vi "Untitled 1.vi"() -> ()   [LabVIEW 2019]
uses:
  Estados.ctl
panel:
  out "HANDLE":u32
  out "Error (\"1\" Error)":bool
  out "Todos":T1(array[cluster])=[{"Device Index"=0, "FT_FLAGS_OPENED"=TRUE, "FT_FLAGS_HISPEED"=TRUE, "Type"=6, "VID"=1027, "PID"=24592, "LocID"=1131585, "Serial Number"="CTAV2022A", "Description"="MI CTA TEST A", "FT_Handle"=433820616}, {"Device Index"=1, "FT_FLAGS_OPENED"=TRUE, "FT_FLAGS_HISPEED"=TRUE, "Type"=6, "VID"=1027, "PID"=24592, "LocID"=1131586, "Serial Number"="CTAV2022B", "Description"="MI CTA TEST B", "FT_Handle"=433822896}]
  out "Array CTA":T1(array[cluster])=[{"Device Index"=0, "FT_FLAGS_OPENED"=TRUE, "FT_FLAGS_HISPEED"=TRUE, "Type"=6, "VID"=1027, "PID"=24592, "LocID"=1131585, "Serial Number"="CTAV2022A", "Description"="MI CTA TEST A", "FT_Handle"=433820616}]
  out "Valor Asic":u16 format="%x"
  in  "error in (no error)":errorcluster
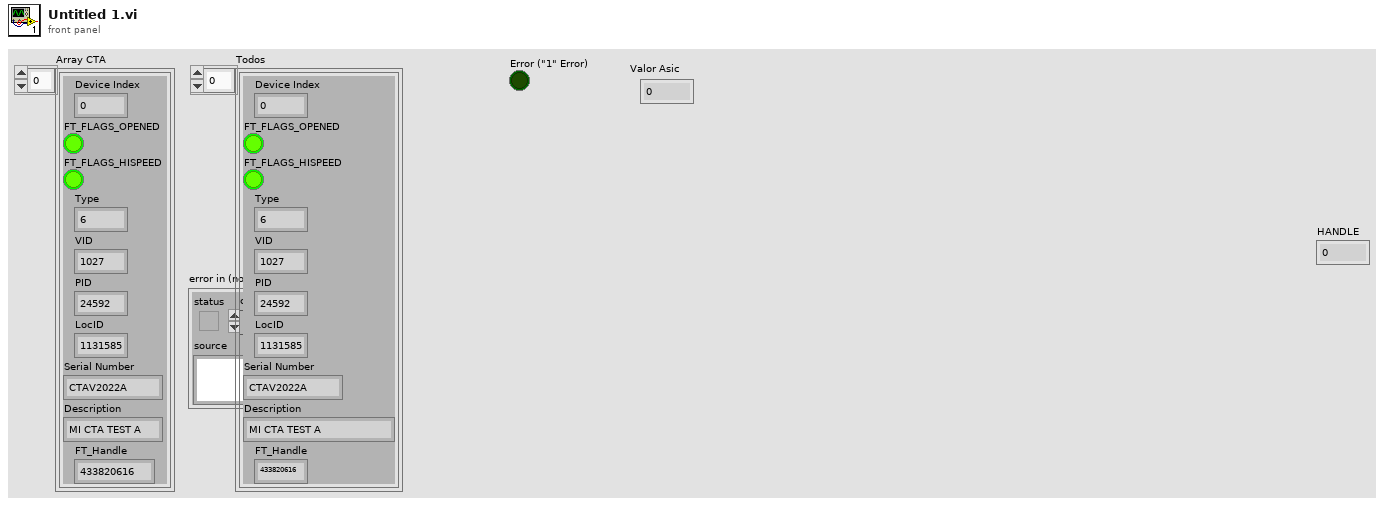
[diagram p1: front panel]
types:
  T1 = cluster{"Device Index":u32, "FT_FLAGS_OPENED":bool, "FT_FLAGS_HISPEED":bool, "Type":u32, "VID":u32, "PID":u32, "LocID":i32, "Serial Number":string, "Description":string, "FT_Handle":u32}[]
  T2 = typedef "Estados.ctl" = enum16{"Inicio", "FuenteON", "Espera", "FuenteOFF", "ObtenerHandle", "InitGen", "Fin", "RateScan", "CerrarVISA"}
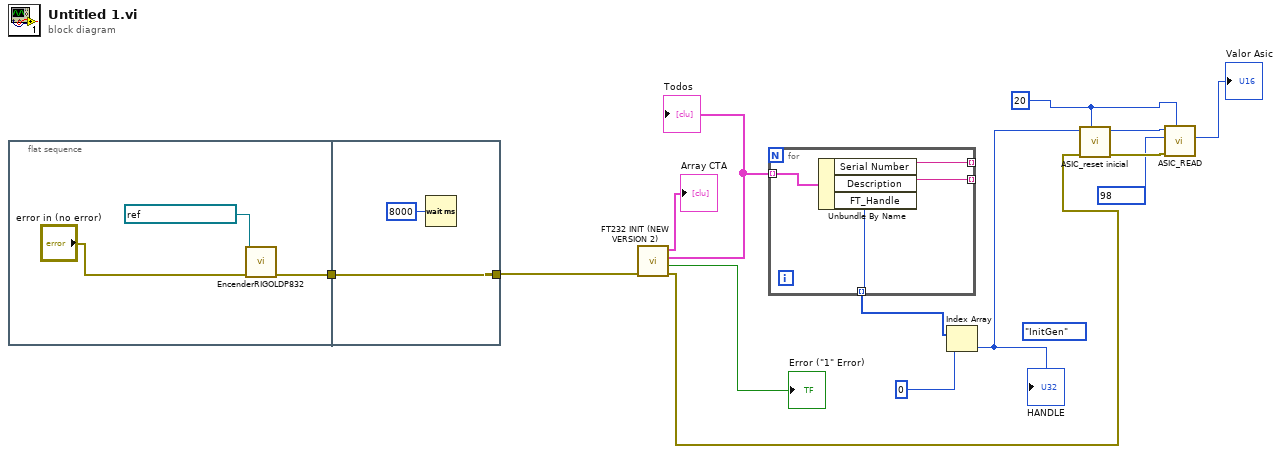
[diagram p0: block diagram]
diagram:
  (unwired) Estados."InitGen"
  w10 = u32 20 ("Espera acceso USB")
  n1 = flat-sequence {
    tunnel: [w15] -> w1
    tunnel: [w19] -> w2
    tunnel: w1 -> [w19]
    frame #0 {
      n2 = call "EncenderRIGOLDP832.vi"("error in (no error)"="error in (no error)", "VISA IN"=refnum<visa-resource-name> "FA_Rigol_DP832") -> ("error out"=w15:errorcluster)  [unwired: 8 in, 1 out]
    }
    frame #1 {
      n3 = Wait (ms)(milliseconds to wait=u32 8000) -> ()  [unwired: 1 out]
    }
  }
  n4 = call "FT232 INIT (NEW VERSION 2).vi"("error in (no error)"=w2) -> ("error out"=w4:errorcluster, "Error (\"1\" Error)"=→"Error (\"1\" Error)":bool, "Todos"=w8:T1, "Array CTA"=→"Array CTA":T1)  [unwired: 7 in]
  "Todos" <- w8
  n5 = for {
    tunnel: w8 -> [w23] mode=indexing
    tunnel: [w22] -> _ mode=indexing
    tunnel: [w21] -> _ mode=indexing
    tunnel: [w20] -> w9 mode=indexing
    n6 = Unbundle By Name(w23) -> ("Serial Number"=w22:string, "Description"=w21:string, "FT_Handle"=w20:u32)
  }
  n7 = Index Array(array=w9, index=0) -> (element=w3:u32)
  "HANDLE" <- w3
  n8 = call "ASIC_reset inicial.vi"("Espera acceso USB"=w10, "error in"=w4, "ftHandle_in"=w3) -> ("error out"=w13:errorcluster, "ftHandle_out"=w14:u32)  [unwired: 7 in]
  n9 = call "ASIC_READ.vi"("Espera acceso USB"=w10, "error in"=w13, "Direccion Registro Asic"=u8 98, "ftHandle_in"=w14) -> ("Valor Asic"=→"Valor Asic":u16)  [unwired: 5 in, 2 out]
